vi "single.vi"(1 "Numeric Input":sgl format="%.2f") -> (0 "Numeric Output":sgl format="%.2f")   [LabVIEW 2011]
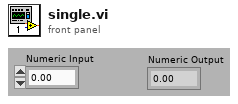
[diagram p1: front panel]
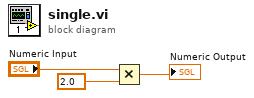
[diagram p0: block diagram]
diagram:
  n1 = Multiply(x="Numeric Input", y=sgl 2.0) -> (x*y=→"Numeric Output":sgl)
